vi "XIPIN_DisplayPort_6_1.vi"   [LabVIEW 2017]
doc: "The DisplayPort Controller is a paramaterizable IP that supports DisplayPort 1.1a and DisplayPort 1.2 features. Support for 1.62 Gbps, 2.7 Gbps and 5.4 Gbps are available as options in the controller. A user can customize the controller to optimize for different bits per color and colorometry. Please refer to product guide for more feature level details.\n------------------------------------\n<b>Need License</b> : Yes\n<b>Interface</b> : AXI4 AXI4-Stream"
uses:
  <vilib>/rvi/XilinxIP/XIPIN_XNode/niFpgaXIPIN.xnode
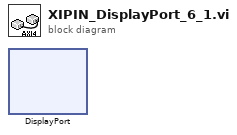
[diagram p0: block diagram]
diagram:
  n1 = xnode ("DisplayPort")() -> ()
